vi "Load MODAQ Configs v2 RD v1.0.vi"(8 "error in (no error)":errorcluster, 10 "MODAQ Config Filename":string="MODAQ Configuration File.xml") -> (0 "error out":errorcluster, 2 "Configs out":T1={"Watch Circle"={"Set Point Lat (dd)"=0.0, "Set Point Lon (dd)"=0.0, "Yellow Alert Radius (m)"=0.0, "Red Alert Radius (m)"=0.0, "AWOL Radius (m)"=0.0, "Yellow Alert Snooze (min)"=0.0, "Red Alert Snooze (min)"=0.0, "AWOL Radius Snooze (min)"=0.0}, "FTP and AWS"={"AWS Access Key"="", "AWS Secret Key"="", "AWS Bucket"="", "Enable AWS Upload (Summary)"=FALSE, "Enable FTP Upload"=FALSE, "FTP Host"="", "FTP User"="", "FTP Password"="", "Destination write path (pos)"="", "Local file path (pos)"="", "Summary  Upload Interval pos (min)"=0, "Delete Local File After Upload"=FALSE, "Destination write path (pow)"="", "Local file path (pow)"="", "Summary Upload Interval pow (min)"=0, "Enable AWS Upload (TDMS)"=FALSE}, "Email Settings"={"Enable Alerts"=FALSE, "Distribution List (comma separated) 1"="", "Distribution List (comma separated) 2"="", "Sender Email"="", "SMTP"="", "Username"="", "Password"=""}, "Summary File"={"Enable CSV"=FALSE, "CSV Averaging Time (Sec)"=0, "CSV Loop Delay (ms)"=0}, "File Settings"={"Config File Path"="", "Data Folder Path"="", "Raw Mode"="", "Raw Interval (min)"=0, "Raw Sampling Time (min)"=0, "TDMS File Write Interval"=enum."10 Min", "Default Filename"=path "MODAQ Configuration File.ini", "Enable TDMS Save (3ph only)"=FALSE}, "Watchdog"={"Watchdog Period (ms)"=1000, "Reset System on WD timeout"=FALSE, "Enable RT Watchdog"=FALSE}, "PowGrp0"={"Channel Names"=["", "", "", "", "", "", "", "", "", "", "", ""], "Channel Units"=["", "", "", "", "", "", "", "", "", "", "", ""], "TDMS File Suffix"="", "Channel Datatype"=["", "", "", "", "", "", "", "", "", "", "", ""]}, "Scaling Factors Grp0"=[], "PowGrp0 Sampling"={"PowGrp0 sample rate [Hz]"=5000.0, "PowGrp0 samples per channel"=500}, "Stbd 3 Phase Voltage Scaling"=[50.0, 50.0, 50.0], "Stbd 3 Phase Current Scaling"=[-12.724, -12.739, -12.73]} {"PowGrp0 Sampling"."PowGrp0 sample rate [Hz]" format="%0.2f"; "Watch Circle"."AWOL Radius Snooze (min)" format="%#_13g"; "Watch Circle"."Red Alert Snooze (min)" format="%#_13g"; "Watch Circle"."Yellow Alert Snooze (min)" format="%#_13g"; "Watch Circle"."AWOL Radius (m)" format="%#_13g"; "Watch Circle"."Red Alert Radius (m)" format="%#_13g"; "Watch Circle"."Yellow Alert Radius (m)" format="%#_13g"; "Watch Circle"."Set Point Lon (dd)" format="%#_13g"; "Watch Circle"."Set Point Lat (dd)" format="%#_13g"})   [LabVIEW 2019]
doc: "Loads the XML configuration file data into a cluster and creates an archive of the loaded XML file that is saved to the Logs folder. The acrchive copy allows for verification of MODAQ settings for a particular run.\n\n2021 NREL"
uses:
  Globals and Definitions/Config Loader TypeDefs/All Tab Controls RDv1.0.ctl
  Globals and Definitions/Config Loader TypeDefs/Watch Circle.ctl
  Globals and Definitions/Config Loader TypeDefs/AWS and FTP.ctl
  Globals and Definitions/Config Loader TypeDefs/Email Settings.ctl
  Globals and Definitions/Config Loader TypeDefs/Summary File.ctl
  Globals and Definitions/Config Loader TypeDefs/File Settings.ctl
  Globals and Definitions/Enum_FileNewInterval.ctl
  Globals and Definitions/Config Loader TypeDefs/Watchdog.ctl
  Globals and Definitions/TDMS Constants.ctl
  <vilib>/Utility/xml.llb/Read From XML File(string).vi
panel:
  # "PT-EN1-1001"
  # "CT-EN1-1001"
  # "PT-EN1-1002"
  # "CT-EN1-1002"
  # "PT-EN1-1003"
  # "CT-EN1-1003"
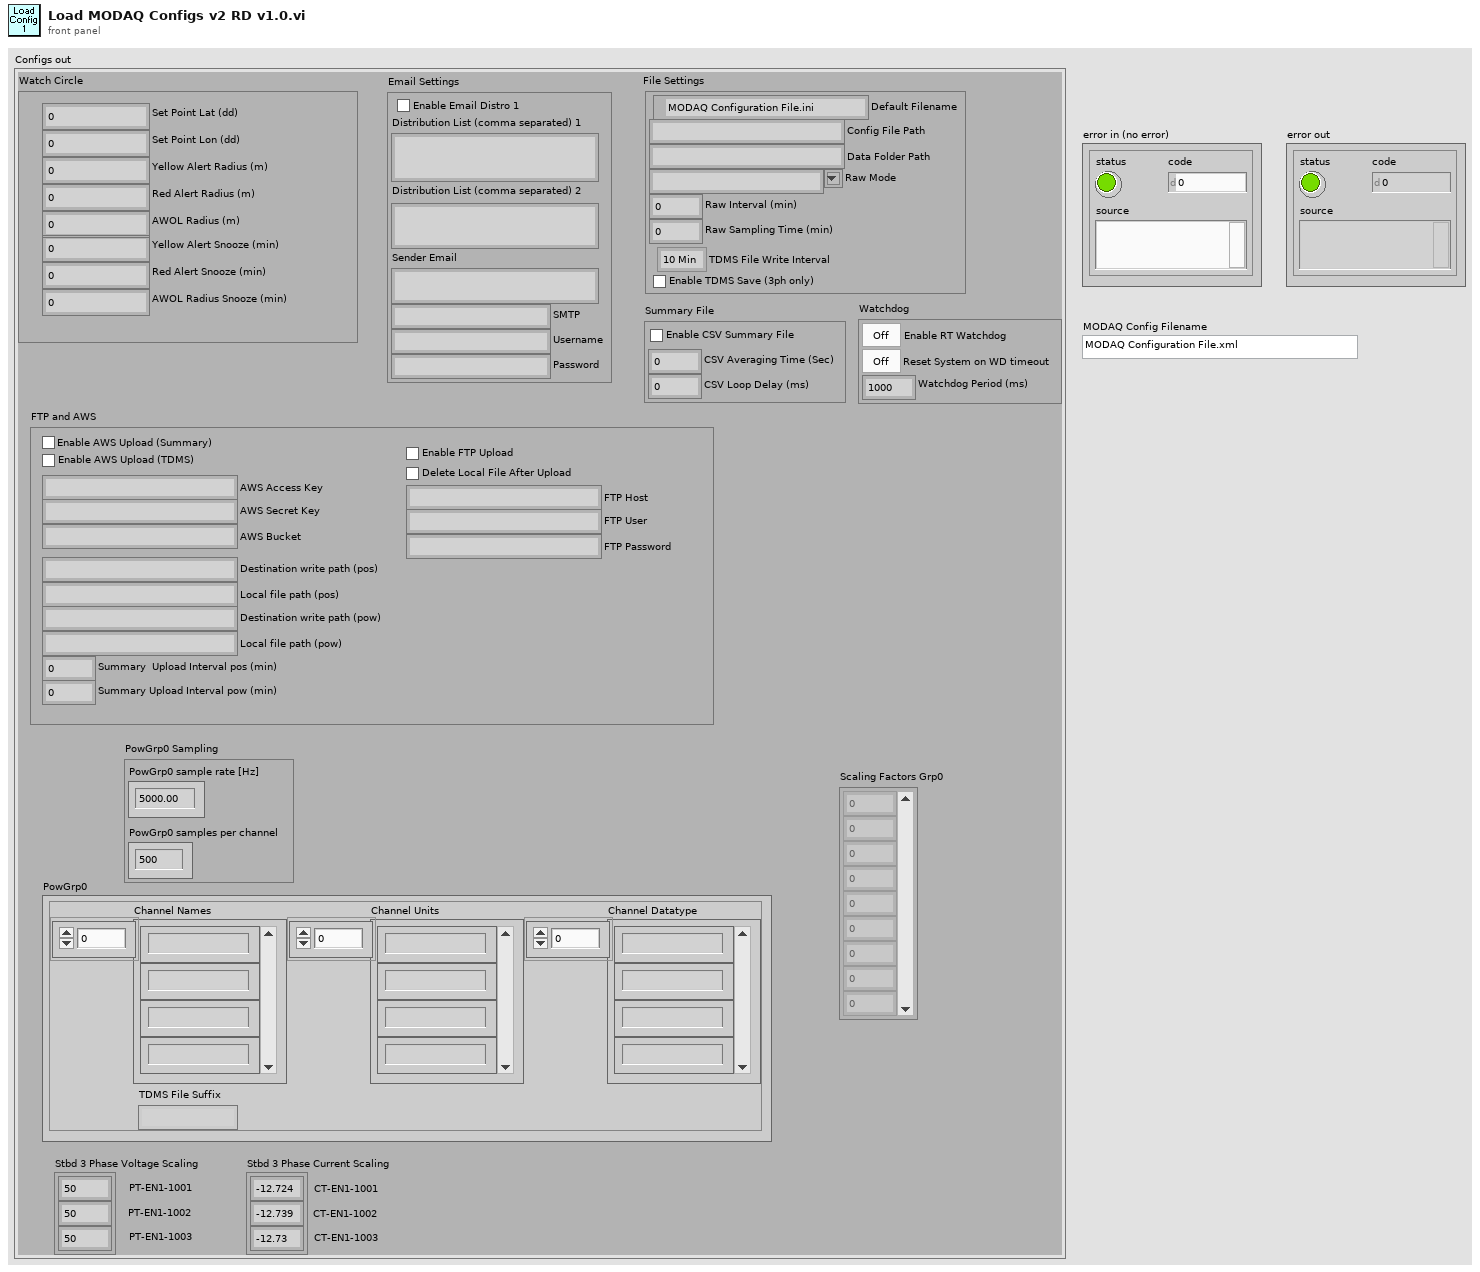
[diagram p1: front panel]
types:
  T1 = typedef "All Tab Controls RDv1.0.ctl" = cluster{"Watch Circle":T2, "FTP and AWS":T3, "Email Settings":T4, "Summary File":T5, "File Settings":T6, "Watchdog":T8, "PowGrp0":T9, "Scaling Factors Grp0":dbl[], "PowGrp0 Sampling":cluster{"PowGrp0 sample rate [Hz]":dbl, "PowGrp0 samples per channel":i32}, "Stbd 3 Phase Voltage Scaling":dbl[], "Stbd 3 Phase Current Scaling":dbl[]}
  T2 = typedef "Watch Circle.ctl" = cluster{"Set Point Lat (dd)":dbl, "Set Point Lon (dd)":dbl, "Yellow Alert Radius (m)":dbl, "Red Alert Radius (m)":dbl, "AWOL Radius (m)":dbl, "Yellow Alert Snooze (min)":dbl, "Red Alert Snooze (min)":dbl, "AWOL Radius Snooze (min)":dbl}
  T3 = typedef "AWS and FTP.ctl" = cluster{"AWS Access Key":string, "AWS Secret Key":string, "AWS Bucket":string, "Enable AWS Upload (Summary)":bool, "Enable FTP Upload":bool, "FTP Host":string, "FTP User":string, "FTP Password":string, "Destination write path (pos)":string, "Local file path (pos)":string, "Summary  Upload Interval pos (min)":i32, "Delete Local File After Upload":bool, "Destination write path (pow)":string, "Local file path (pow)":string, "Summary Upload Interval pow (min)":i32, "Enable AWS Upload (TDMS)":bool}
  T4 = typedef "Email Settings.ctl" = cluster{"Enable Alerts":bool, "Distribution List (comma separated) 1":string, "Distribution List (comma separated) 2":string, "Sender Email":string, "SMTP":string, "Username":string, "Password":string}
  T5 = typedef "Summary File.ctl" = cluster{"Enable CSV":bool, "CSV Averaging Time (Sec)":i32, "CSV Loop Delay (ms)":i32}
  T6 = typedef "File Settings.ctl" = cluster{"Config File Path":string, "Data Folder Path":string, "Raw Mode":string, "Raw Interval (min)":i32, "Raw Sampling Time (min)":i32, "TDMS File Write Interval":T7, "Default Filename":path, "Enable TDMS Save (3ph only)":bool}
  T7 = typedef "Enum_FileNewInterval.ctl" = enum16{"10 Min", "Hourly", "Daily", "Weekly", "Monthly"}
  T8 = typedef "Watchdog.ctl" = cluster{"Watchdog Period (ms)":u32, "Reset System on WD timeout":bool, "Enable RT Watchdog":bool}
  T9 = typedef "TDMS Constants.ctl" = cluster{"Channel Names":string[], "Channel Units":string[], "TDMS File Suffix":string, "Channel Datatype":string[]}
  T10 = typedef "LVDateTimeRec.ctl" = cluster{"fractional second":dbl, "second":i32, "minute":i32, "hour":i32, "day of month":i32, "month":i32, "year":i32, "day of week":i32, "day of year":i32, "DST":i32}
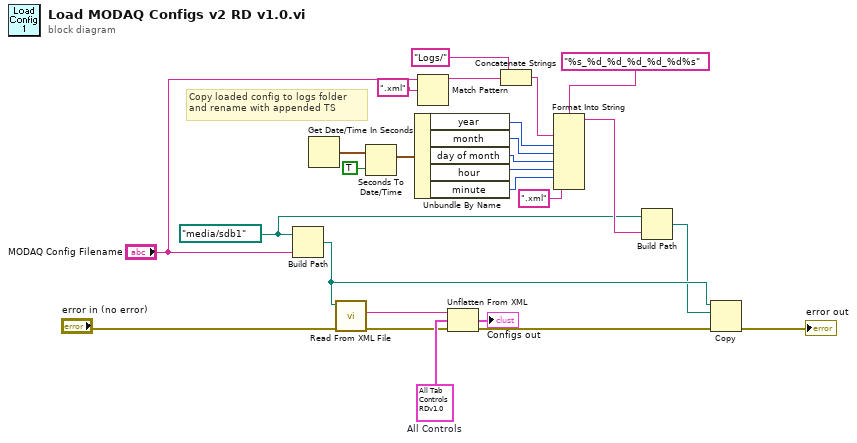
[diagram p0: block diagram]
diagram:
  w25 = T1 {"Watch Circle"={"Set Point Lat (dd)"=0.0, "Set Point Lon (dd)"=0.0, "Yellow Alert Radius (m)"=0.0, "Red Alert Radius (m)"=0.0, "AWOL Radius (m)"=0.0, "Yellow Alert Snooze (min)"=0.0, "Red Alert Snooze (min)"=0.0, "AWOL Radius Snooze (min)"=0.0}, "FTP and AWS"={"AWS Access Key"="", "AWS Secret Key"="", "AWS Bucket"="", "Enable AWS Upload (Summary)"=FALSE, "Enable FTP Upload"=FALSE, "FTP Host"="", "FTP User"="", "FTP Password"="", "Destination write path (pos)"="", "Local file path (pos)"="", "Summary  Upload Interval pos (min)"=0, "Delete Local File After Upload"=FALSE, "Destination write path (pow)"="", "Local file path (pow)"="", "Summary Upload Interval pow (min)"=0, "Enable AWS Upload (TDMS)"=FALSE}, "Email Settings"={"Enable Alerts"=FALSE, "Distribution List (comma separated) 1"="", "Distribution List (comma separated) 2"="", "Sender Email"="", "SMTP"="", "Username"="", "Password"=""}, "Summary File"={"Enable CSV"=FALSE, "CSV Averaging Time (Sec)"=0, "CSV Loop Delay (ms)"=0}, "File Settings"={"Config File Path"="", "Data Folder Path"="", "Raw Mode"="", "Raw Interval (min)"=0, "Raw Sampling Time (min)"=0, "TDMS File Write Interval"=enum."10 Min", "Default Filename"=path "", "Enable TDMS Save (3ph only)"=FALSE}, "Watchdog"={"Watchdog Period (ms)"=0, "Reset System on WD timeout"=FALSE, "Enable RT Watchdog"=FALSE}, "PowGrp0"={"Channel Names"=["CT-EN6-2003", "CT-EN6-3001", "CT-EN6-3002", "PT-EN6-1001", "CT-EN1-1005", "CT-EN2-1005", "CT-EN6-2001", "CT-EN6-2002", "PT-EN6-1002", "CT-EN7-1001", "PT-EN7-1001", "TimeStamp"], "Channel Units"=["ADC", "ADC", "ADC", "VDC", "ADC", "ADC", "ADC", "ADC", "VDC", "ADC", "VDC", "UTC"], "TDMS File Suffix"="PowGrp2", "Channel Datatype"=["Float", "Float", "Float", "Float", "Float", "Float", "Float", "Float", "Float", "Float", "Float", "Float"]}, "Scaling Factors Grp0"=[], "PowGrp0 Sampling"={"PowGrp0 sample rate [Hz]"=5000.0, "PowGrp0 samples per channel"=500}, "Stbd 3 Phase Voltage Scaling"=[50.0, 50.0, 50.0], "Stbd 3 Phase Current Scaling"=[-12.724, -12.739, -12.73]}  # All Controls
  w6 = path "/media/sdb1" ("Config file path")
  # "Copy loaded config to logs folder\nand rename with appended TS"
  n1 = Build Path(base path=w6, name or relative path="MODAQ Config Filename") -> (appended path=w20:path)
  n2 = Get Date/Time In Seconds() -> (seconds since 1Jan1904=w12:timestamp)
  n3 = call-poly <vilib>:"Read From XML File.vi"("error in (no error)"="error in (no error)", "XML File Path"=w20) -> ("error out"=w23:errorcluster, "XML Elements"=w26:string)  [unwired: 7 in, 1 out]
  n4 = Seconds To Date/Time(time stamp (now)=w12, to UTC (F)=TRUE) -> (date time rec=w19:T10)
  n5 = Unbundle By Name(w19) -> ("year"=w17:i32, "month"=w16:i32, "day of month"=w15:i32, "hour"=w14:i32, "minute"=w13:i32)
  n6 = Match Pattern(string="MODAQ Config Filename", regular expression=".xml") -> (before substring=w9:string)  [unwired: 1 in, 3 out]
  n7 = Unflatten From XML(xml string=w26, type=w25, error in (no error)=w23) -> (value=→"Configs out":T1, error out=w22:errorcluster)
  n8 = Concatenate Strings("Logs/" ("input 1"), w9) -> (w8:string)
  n9 = Format Into String(format string="%s_%d_%d_%d_%d_%d%s", w8, w17, w16, w15, w14, w13, ".xml" ("name or relative path")) -> (resulting string=w7:string)  [unwired: 2 in, 1 out]
  n10 = Build Path(base path=w6, name or relative path=w7) -> (appended path=w5:path)
  n11 = Copy(8:w22, 10:w5, 11:w20) -> (0:→"error out":errorcluster)  [unwired: 2 in, 2 out]
